vi "sub_dir_filter.vi"(10 "speed":i16, 11 "set_pt":i16) -> (3 "ok":bool)   [LabVIEW 2018]
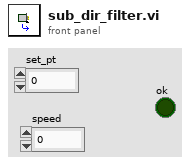
[diagram p1: front panel]
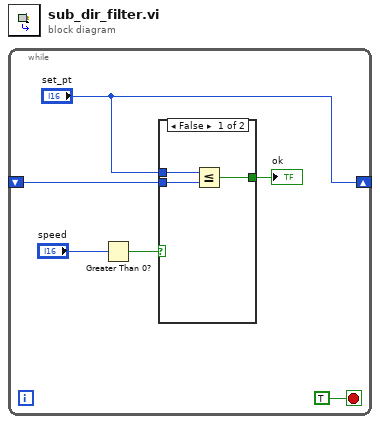
[diagram p0: block diagram]
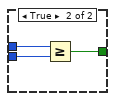
[diagram p2: hidden frame]
diagram:
  n1 = while {
    shift-right: ["set_pt"] -> _
    shift-left: _ -> [w2]
    stop <- TRUE stop-if-true
    n2 = Greater Than 0?(x="speed") -> (x > 0?=w4:bool)
    n3 = case shown="False" w4 {
      tunnel: "set_pt" -> [w7 w12]
      tunnel: w2 -> [w8 w11]
      tunnel: [w9 w10] -> w1
      frame False {
        n4 = Less Or Equal?(x=w7, y=w8) -> (x <= y?=w9:bool)
      }
      frame True {
        n5 = Greater Or Equal?(x=w12, y=w11) -> (x >= y?=w10:bool)
      }
    }
    "ok" <- w1
  }
